vi "Reset Power.vi"(8 "error in (no error)":errorcluster, 10 "Wavelengths":u16[](array[numeric]), 11 "Laser in":refnum<class "Laser.lvclass">) -> (0 "error out":errorcluster, 3 "Laser out":refnum<class "Laser.lvclass">)   [LabVIEW 2018, in "Laser.lvlib" / "Laser.lvclass"]
uses:
  Laser.lvclass
  Laser.lvclass/Laser.ctl
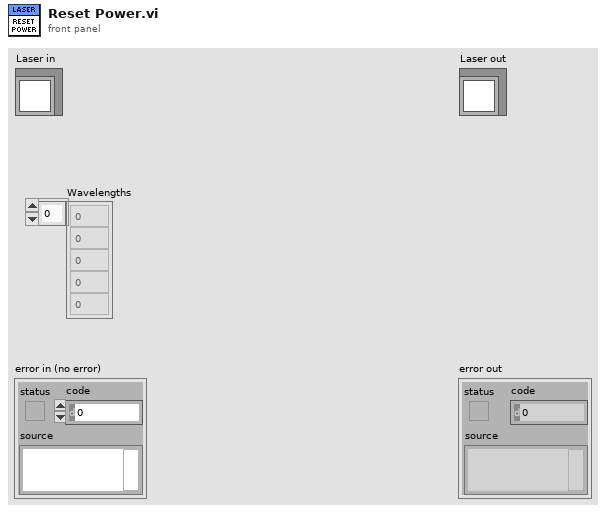
[diagram p1: front panel]
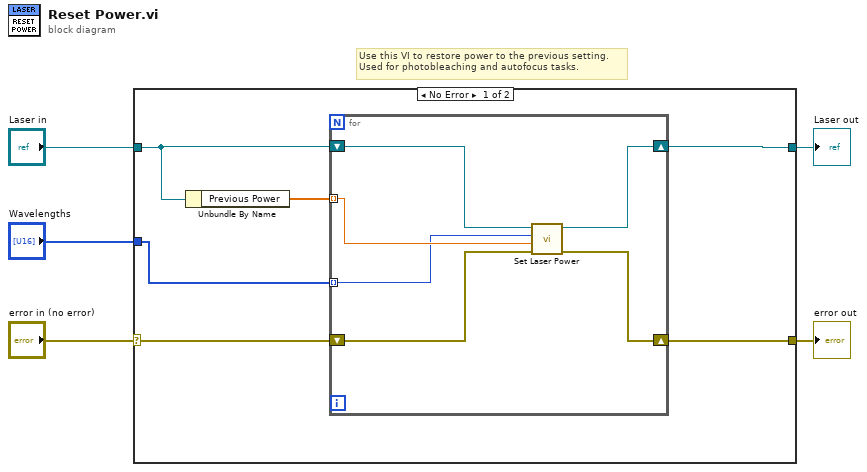
[diagram p0: block diagram]
diagram:
  # "Use this VI to restore power to the previous setting.\nUsed for photobleaching and autofocus tasks."
  n1 = case shown="No Error" "error in (no error)" {
    selector: "error in (no error)" -> [w9 w19]
    tunnel: [w8 w19] -> w4
    tunnel: [w10 w18] -> w2
    tunnel: "Laser in" -> [w11 w18]
    tunnel: "Wavelengths" -> [w6 _]
    frame No Error {
      n2 = Unbundle By Name(w11) -> ("Previous Power"=w7:dbl[])
      n3 = for {
        shift-right: [w16] -> w10
        shift-left: w11 -> [w17]
        shift-right: [w14] -> w8
        shift-left: w9 -> [w15]
        tunnel: w7 -> [w13] mode=indexing
        tunnel: w6 -> [w12] mode=indexing
        n4 = call-dynamic "Set Laser Power.vi"("error in (no error)"=w15, "Power"=w13, "Wavelength"=w12, "Laser Quantum in"=w17) -> ("error out"=w14:errorcluster, "Laser Quantum out"=w16:refnum<class "Laser.lvclass">)  [unwired: 6 in]
      }
    }
    frame Error {
    }
  }
  "error out" <- w4
  "Laser out" <- w2
